vi "STAGE+mono+counter_edit18.vi"() -> ()   [LabVIEW 2017]
panel:
  out "Array 3":dbl[][](array[numeric])
  out "Array 2":dbl[](array[numeric])
  out "XY Graph 2":cluster{dbl[], dbl[]}[](graph)
  out "Waveform Graph":waveform(dbl)[](graph)
  out "XY Graph":cluster{dbl[], dbl[]}(graph)
  out "PROGRESS":u8(slide) max=10 step=10 scale=0.0..5.0
  in  "?":enum32{"DELAY", "COUNTER", "MONO", "PLOT"}(tab)
  out "Final time [ps]":dbl
  out "Current time [ps]":dbl
  out "Initial time [ps]":dbl
  in  "Set this as t0":bool
  in  "Axis":i32=1
  in  "Motor ON":bool
  in  "Motor OFF":bool
  out "Current Position [mm]":dbl
  out "Final Position [mm]":dbl
  in  "Data Points":i32=100
  out "Current Point":i32
  in  "Step Size [um]":i32=10
  in  "Target [mm]":dbl format="%.3f"
  in  "Move":bool
  out "Initial position [mm]":dbl
  in  "GPIB address":string="23"
  in  "Count Mode":u16(ring) items=["A,B for Preset T", "A-B for Preset T", "A+B for Preset T", "A for Preset B"]
  in  "Trigger mode":u16(ring) items=["10 MHz"=0, "Input 2"=2, "Input T"=3]
  in  "Channel A Input":u16(ring)=1 items=["10 MHz", "Input 1"]
  in  "Channel B Input":u16(ring)=2 items=["Input 1"=1, "Input 2"=2]
  in  "Number of Measurements\n to take at one point/ Number of Periods":u16=1 min=1 max=2000 step=1
  in  "Time between measurements\n at one point (s)/Dwell Time":dbl=0.002 min=0.002 max=60.0 step=0.001
  in  "gate mode (CW:0)":i16(slide) scale=0.0..2.0 scale format="%.2f"
  out "Counts":i32
  in  "Integrating time \nin 10^-7 sec":dbl=10000000.0
  in  "Discriminator Level (mV)":dbl min=-300.0 max=300.0 step=0.2
  in  "Discriminator Slope":bool
  in  "Channel":i16 min=0 max=2 step=1
  out "Grating #":dbl
  out "Blaze angle":dbl
  out "Grooves/mm":dbl
  out "Mono port":T1(ring)
  out "Time delay":u32=450000 min=1
  in  "Step size":dbl=10.0 min=0.0
  in  "Scan to":i32=4000
  in  "Scan from":i32=2600
  out "Current wavelength":dbl
  in  "?":bool
  in  "Array":dbl[](array[numeric])
  out "Numeric":i32
  out "Numeric 2":i32
  out "Timeout 2":bool
  in  "?":bool
  out "Timeout":bool
  in  "Collect Data!":bool
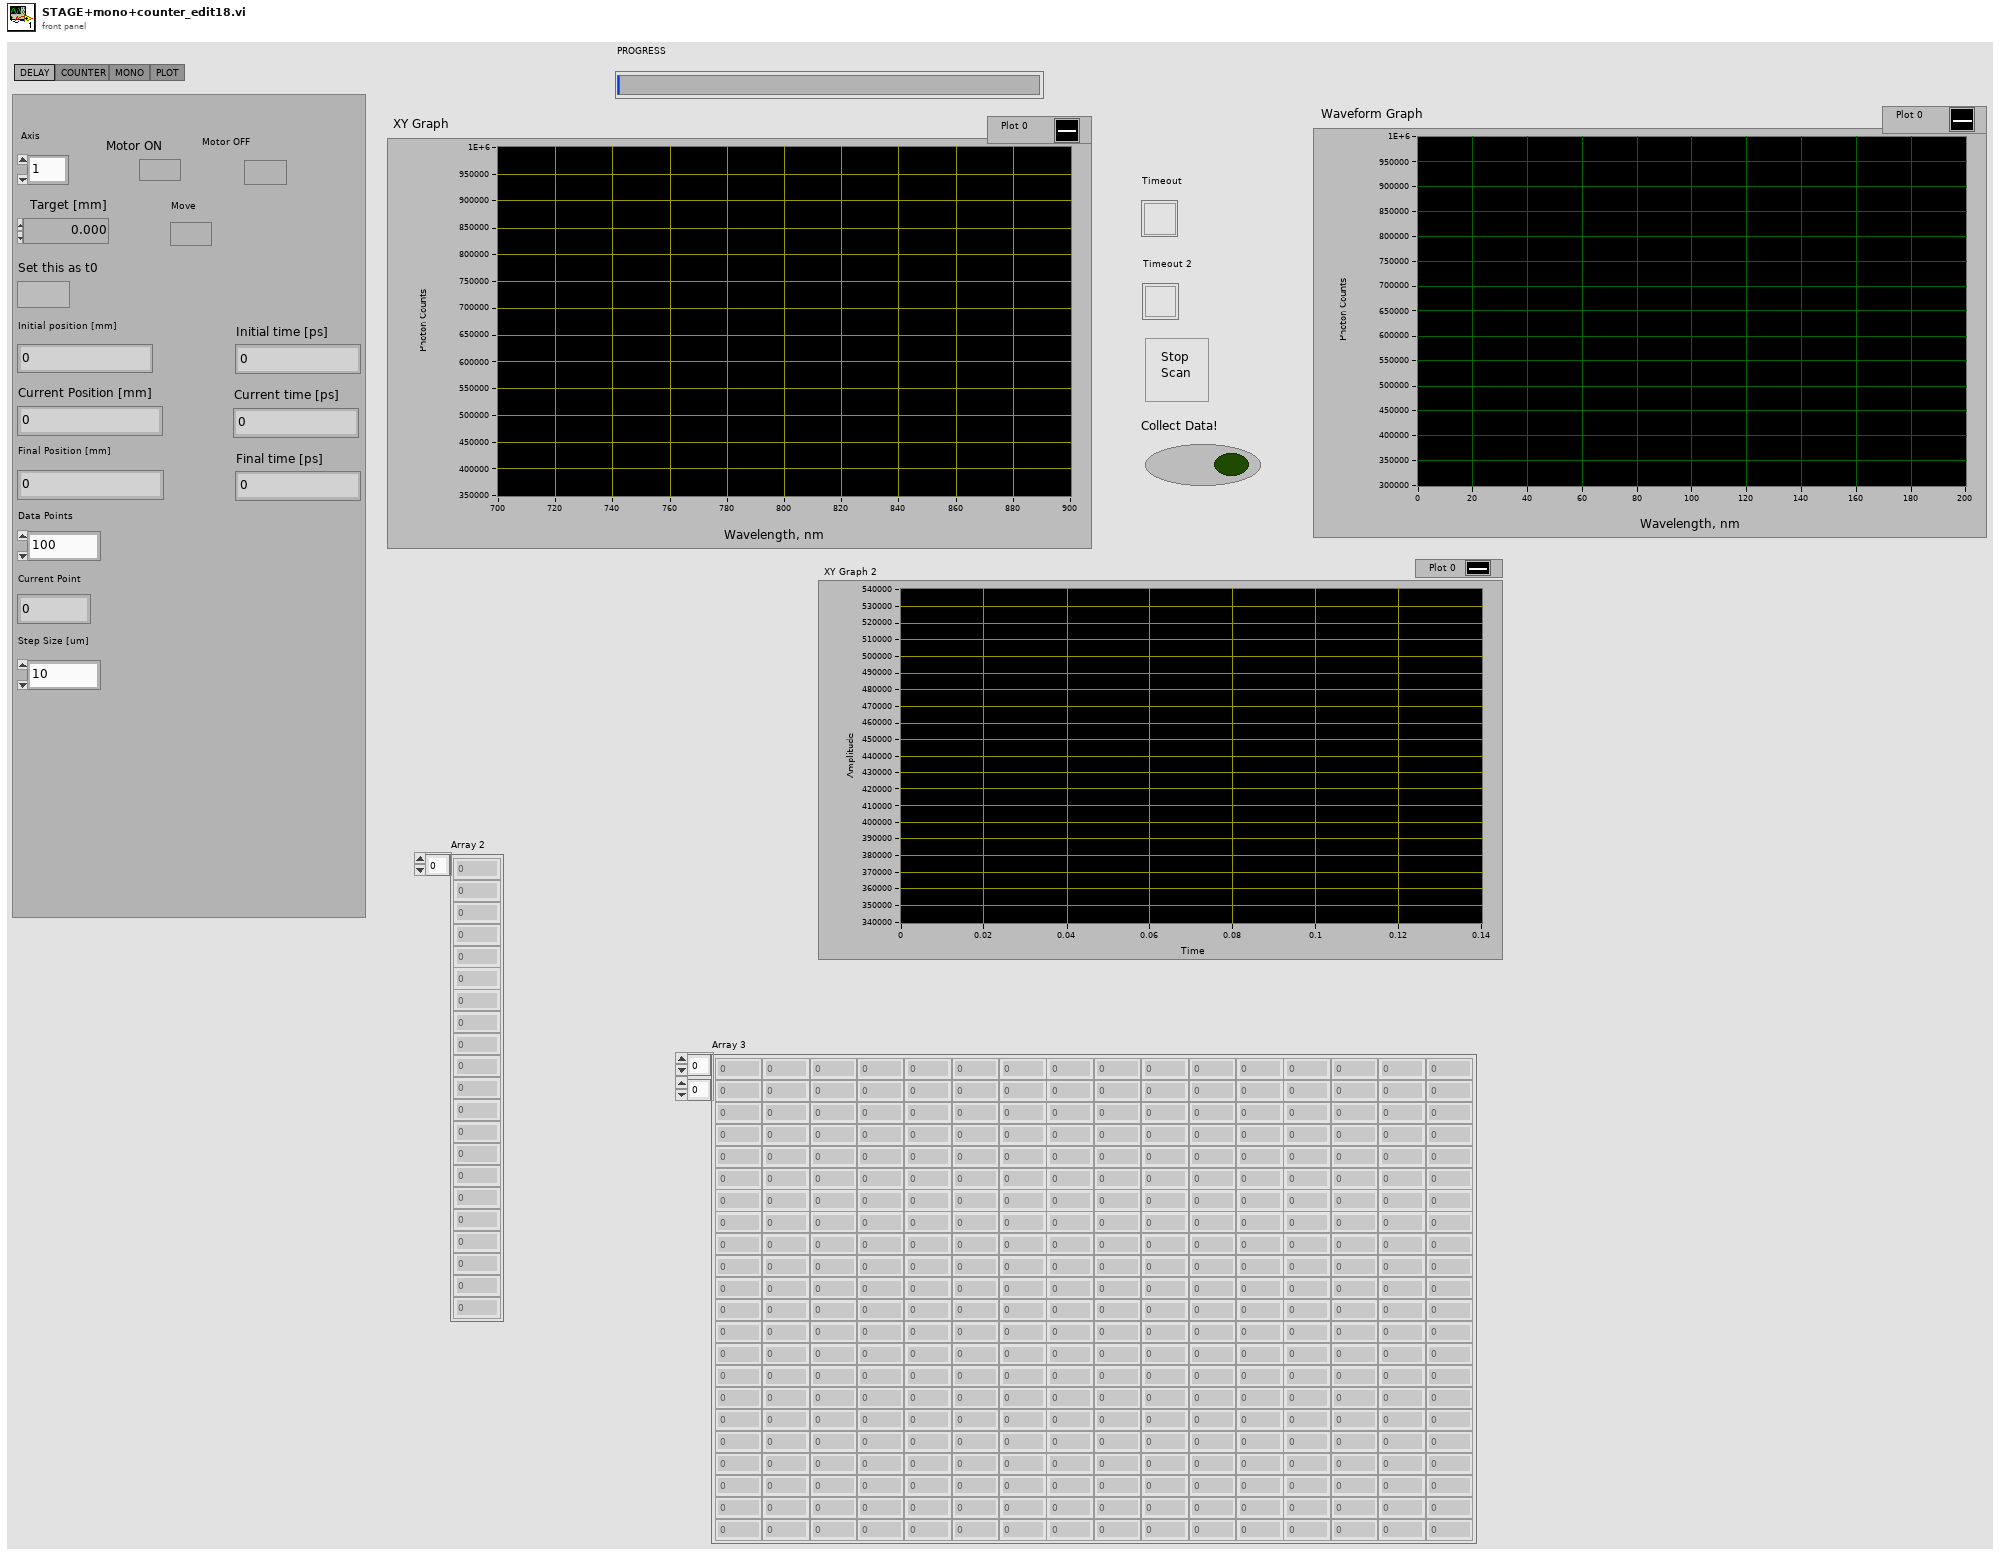
[diagram p1: front panel]
types:
  T1 = enum8{"COM 1", "COM 2", "COM 3", "COM 4", "COM 5", "COM 6", "COM 7", "COM 8", "COM 9"}
  T2 = cluster{"input XON/XOFF":bool, "input HW Handshake":bool, "input alt HW HShk":bool, "output XON/XOFF":bool, "output HW Handshake":bool, "output alt HW HShk":bool, "XOFF byte":u8, "XON byte":u8, "parity error byte":u16}
  T3 = enum16{"no parity", "odd parity", "even parity", "mark parity", "space parity"}
  T4 = typedef "NI_Matrix.lvlib/RealMatrix.ctl" = dbl[][]
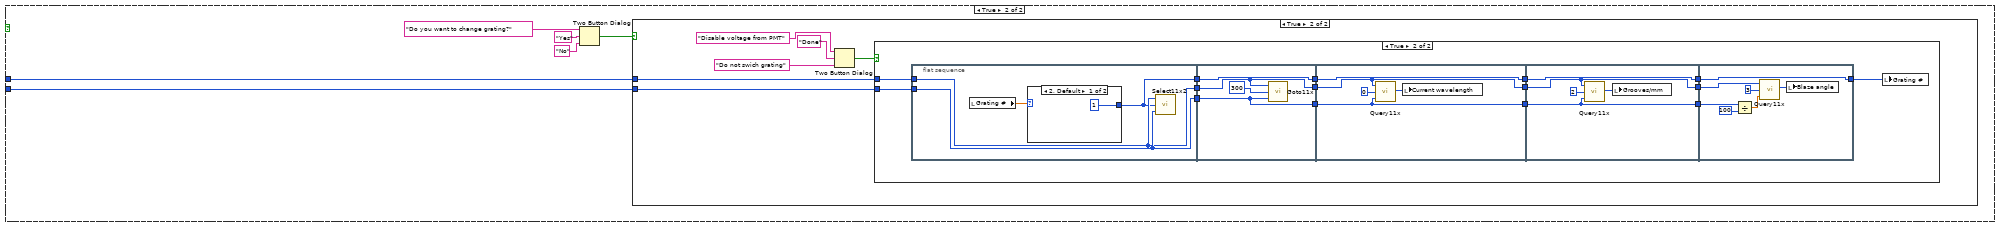
[diagram p2: hidden frame]
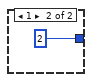
[diagram p5: hidden frame]
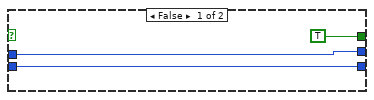
[diagram p6: hidden frame]
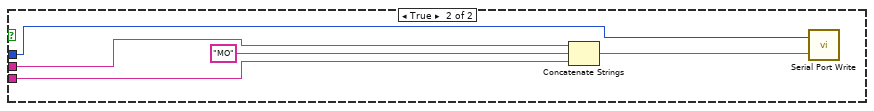
[diagram p7: hidden frame]
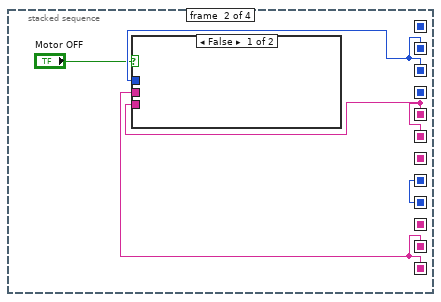
[diagram p8: hidden frame]
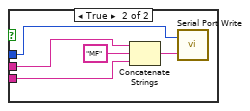
[diagram p9: hidden frame]
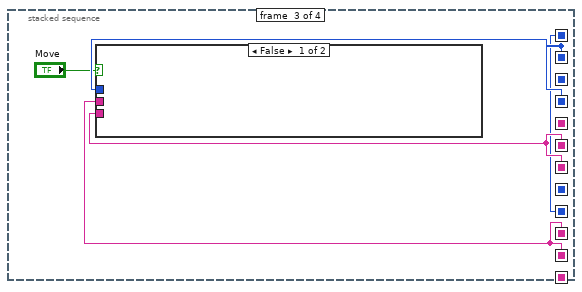
[diagram p10: hidden frame]
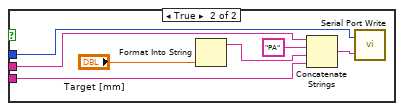
[diagram p11: hidden frame]
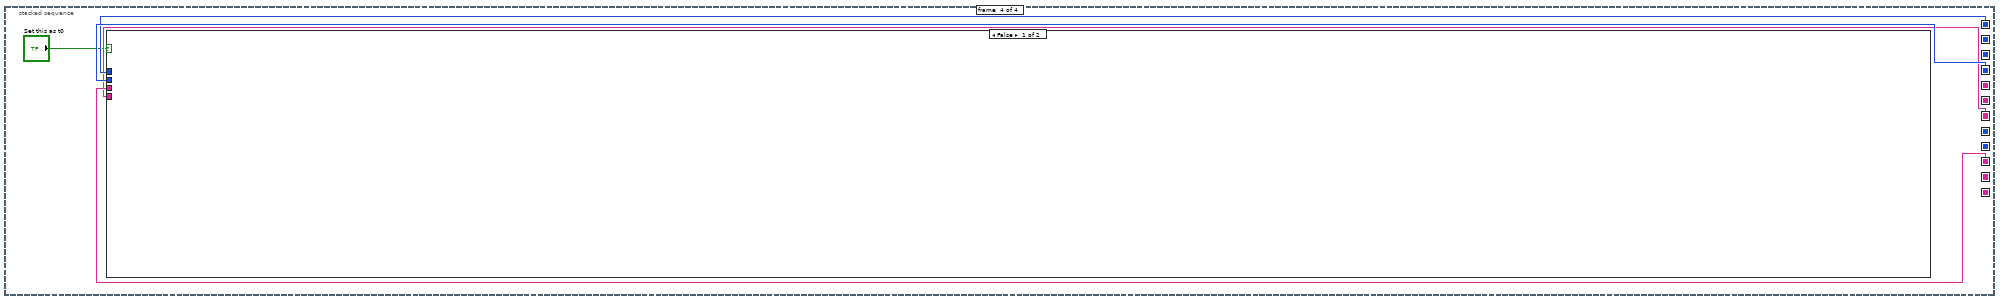
[diagram p12: hidden frame]
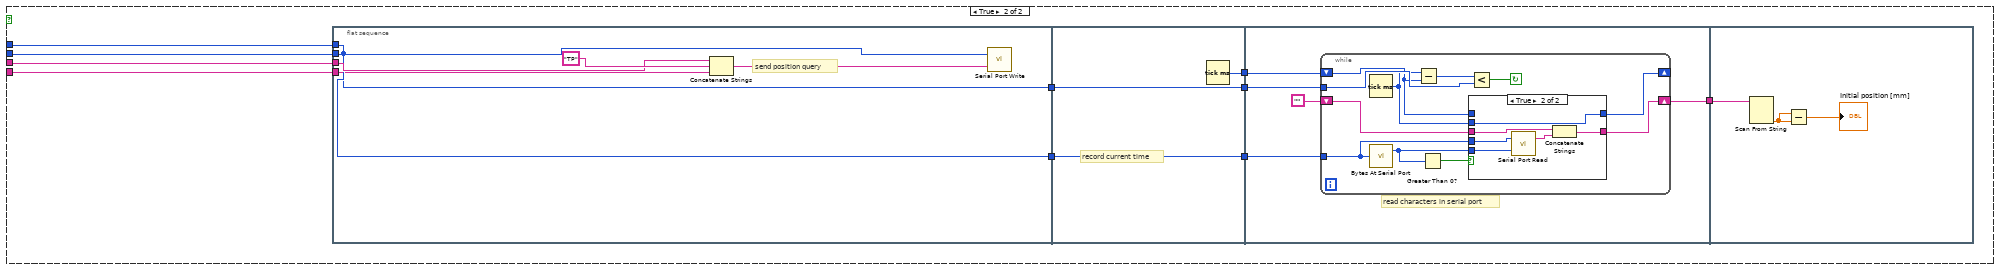
[diagram p13: hidden frame]
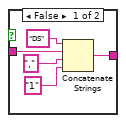
[diagram p15: hidden frame]
diagram:
  (unwired) FALSE
  w41 = u32 19200  # baud rate
  w40 = u16 8  # data bits
  w39 = enum16{"1 bit", "1.5 bits", "2 bits"}."1 bit"  # stop bits
  w43 = T3."no parity"  # parity
  w38 = 4  # 0=COM1 so n=COM(n+1)
  w42 = u16 1024  # buffer size
  n1 = flat-sequence {
    tunnel: ["Data Points"] -> w47
    tunnel: "Axis" -> [w69]
    tunnel: [w61] -> w46
    tunnel: [w69] -> w45
    tunnel: ["Step Size [um]"] -> w19
    tunnel: [w61] -> w18
    tunnel: ["Step Size [um]"] -> w17
    tunnel: ["Data Points"] -> w16
    tunnel: [w61] -> w15
    tunnel: [w60] -> w14
    tunnel: [w61] -> w12
    tunnel: [w60] -> w11
    tunnel: [w63] -> w10
    tunnel: [w52] -> w9
    tunnel: [w53] -> w2
    tunnel: [w52] -> w1
    tunnel: w47 -> [w158]
    tunnel: w46 -> [w157]
    tunnel: w45 -> [w156]
    tunnel: w38 -> [w152]
    tunnel: "GPIB address" -> [w151]
    tunnel: "GPIB address" -> [w150]
    tunnel: w19 -> [w139]
    tunnel: w18 -> [w137]
    tunnel: w17 -> [w136]
    tunnel: w16 -> [w134]
    tunnel: w15 -> [w129]
    tunnel: w14 -> [w128]
    tunnel: "Integrating time \nin 10^-7 sec" -> [w127]
    tunnel: w12 -> [w125]
    tunnel: w11 -> [w124]
    tunnel: w10 -> [w123]
    tunnel: w9 -> [w121]
    tunnel: w5 -> [w111]
    tunnel: w4 -> [w110]
    tunnel: w3 -> [w109]
    tunnel: w2 -> [w77]
    tunnel: w1 -> [w76]
    frame #0 {
      n2 = while {
        stop <- "Collect Data!" stop-if-true
        n3 = Multiply(x=1, y=1000) -> (x*y=w51:i32)
        n4 = Wait (ms)(milliseconds to wait=w51) -> ()  [unwired: 1 out]
      }
    }
    frame #1 {
      w54 = 1000000000000.0
      w59 = 1000
      w62 = 300000000
      w64 = 1000
      n5 = local read "Initial position [mm]"() -> (w61:dbl)
      n6 = Multiply(x="Step Size [um]", y="Data Points") -> (x*y=w68:i32)
      n7 = Divide(x="Step Size [um]", y=w64) -> (x/y=w63:dbl)
      n8 = Divide(x=w68, y=w64) -> (x/y=w67:dbl)
      n9 = Add(x=w61, y=w67) -> (x+y=w60:dbl)
      "Final Position [mm]" <- w60
      n10 = Divide(x=w60, y=w59) -> (x/y=w58:dbl)
      n11 = Divide(x=w61, y=w59) -> (x/y=w57:dbl)
      n12 = Divide(x=w58, y=w62) -> (x/y=w55:dbl)
      n13 = Divide(x=w57, y=w62) -> (x/y=w56:dbl)
      n14 = Multiply(x=w55, y=w54) -> (x*y=w53:dbl)
      "Final time [ps]" <- w53
      n15 = Multiply(x=w56, y=w54) -> (x*y=w52:dbl)
      "Initial time [ps]" <- w52
    }
    frame #2 {
      w91 = "\r\n"
      n16 = Increment(x=w134) -> (x+1=w135:i32)
      n17 = Divide(x=w139, y=1000.0) -> (x/y=w115:dbl)
      n18 = for {
        N: w135 -> [_]
        tunnel: w115 -> [w169]
        tunnel: w137 -> [w167]
        tunnel: [w160] -> w133 mode=indexing
        i -> [w168]
        # "distances"
        n19 = Multiply(x=w169, y=w168) -> (x*y=w166:dbl)
        n20 = Add(x=w167, y=w166) -> (x+y=w165:dbl)
        n21 = Divide(x=w165, y=1000) -> (x/y=w159:dbl)
        n22 = Divide(x=w159, y=300000000) -> (x/y=w162:dbl)
        n23 = Multiply(x=w162, y=1000000000000.0) -> (x*y=w160:dbl)
      }
      n24 = To Time Stamp(1:"Scan from") -> (0:w82:timestamp)
      n25 = Multiply(x="Scan to", y=1) -> (x*y=w122:i32)
      n26 = Multiply(x=1, y="Scan from") -> (x*y=w114:i32)
      n27 = Divide(x=w115, y=1000.0) -> (x/y=w116:dbl)
      n28 = Subtract(x=w122, y=w114) -> (x-y=w145:i32)
      n29 = Divide(x=w145, y="Step size") -> (x/y=w144:dbl)
      n30 = Divide(x=w116, y=300000000) -> (x/y=w118:dbl)
      n31 = Bundle By Name("Y"=dbl[] [], "t0"=w82, "dt"="Step size") -> (w79:waveform(dbl))  [unwired: 1 in]
      n32 = local read "Numeric"() -> (w71:i32)
      n33 = Multiply(x=w118, y=1000000000000.0) -> (x*y=w75:dbl)
      n34 = local read "Numeric 2"() -> (w72:i32)
      n35 = Build Array(w79) -> (w78:waveform(dbl)[])
      n36 = Round Toward -Infinity(1:w144) -> (0:w143:dbl)
      n37 = Concatenate Strings("\r", "\n") -> (w153:string)
      n38 = property on="XY Graph 2" class="XYGraph (strict)"("XScale.Increment"=w75, "XScale.Maximum"=w77, "XScale.Minimum"=w76) -> ()  [unwired: 2 in, 2 out]
      n39 = Initialize Array(0.0, w71, w72) -> ()  [unwired: 1 out]
      n40 = Increment(x=w143) -> (x+1=w113:dbl)
      n41 = for {
        N: w158 -> [w184]
        tunnel: w157 -> [w247]
        tunnel: w136 -> [w243]
        tunnel: w156 -> [w240]
        tunnel: w153 -> [w237]
        tunnel: w152 -> [w238]
        tunnel: w151 -> [w236]
        tunnel: w110 -> [w233]
        tunnel: w111 -> [w235]
        tunnel: w150 -> [w234]
        tunnel: [w194] -> w84 mode=indexing
        tunnel: w114 -> [w228]
        tunnel: "Step size" -> [w227]
        tunnel: w143 -> [w226]
        tunnel: w129 -> [_]
        tunnel: w128 -> [_]
        tunnel: w127 -> [w225]
        tunnel: "Scan to" -> [w224]
        tunnel: "Scan from" -> [w223]
        tunnel: "Step size" -> [w200]
        tunnel: w125 -> [w216]
        tunnel: w124 -> [w214]
        tunnel: w123 -> [w217]
        tunnel: w75 -> [w186]
        tunnel: w121 -> [w221]
        tunnel: "Scan from" -> [w201]
        tunnel: "Step size" -> [w202]
        shift-right: [w185] -> _
        shift-left: dbl[] [] -> [w180]
        tunnel: w111 -> [w199]
        tunnel: w110 -> [w198]
        tunnel: w109 -> [w197]
        shift-right: [w191] -> _
        shift-left: w78 -> [w192]
        shift-right: [w178] -> _
        shift-left: dbl[][] [] -> [w177]
        i -> [w183]
        w196 = dbl[] []
        w215 = 1000
        w218 = 300000000
        n42 = To Time Stamp(1:w228) -> ()  [unwired: 1 out]
        n43 = property on="PROGRESS" class="Slide (strict)"("Scale.Increment"=1, "Scale.Maximum"=w184, "Scale.Minimum"=0) -> ()  [unwired: 2 in, 2 out]
        n44 = flat-sequence {
          tunnel: w236 -> [w273]
          tunnel: w235 -> [w272]
          tunnel: w233 -> [w271]
          tunnel: w228 -> [w270]
          tunnel: w227 -> [w269]
          tunnel: w226 -> [w268]
          tunnel: w224 -> [w267]
          tunnel: w223 -> [w266]
          tunnel: w196 -> [w265]
          tunnel: w196 -> [w264]
          tunnel: w202 -> [w263]
          tunnel: w201 -> [w262]
          tunnel: w200 -> [w261]
          tunnel: w199 -> [w260]
          tunnel: w198 -> [w259]
          tunnel: w197 -> [w258]
          tunnel: [w256] -> w195
          tunnel: [w257] -> _
          tunnel: [w256] -> w193
          tunnel: [w438] -> w194
          tunnel: w195 -> [w438]
          tunnel: [w437] -> w179
          tunnel: [w436] -> w176
          frame #0 {
            # "step size"
            n45 = while {
              tunnel: w271 -> [_]
              tunnel: w272 -> [_]
              tunnel: w273 -> [w279]
              tunnel: w270 -> [w307]
              tunnel: w269 -> [w306]
              tunnel: w268 -> [w305]
              tunnel: w267 -> [w275]
              tunnel: w266 -> [w274]
              tunnel: w261 -> [w276]
              tunnel: w263 -> [w303]
              shift-right: [w299] -> w256
              shift-left: w264 -> [w298]
              shift-right: [w293] -> w257
              shift-left: w265 -> [w301]
              tunnel: w262 -> [w296]
              tunnel: w260 -> [w283]
              tunnel: w259 -> [w282]
              tunnel: w258 -> [w281]
              i -> [w304]
              stop <- w310 stop-if-true
              n46 = property on="XY Graph" class="XYGraph (strict)"("XScale.Increment"=w276, "XScale.Maximum"=w275, "XScale.Minimum"=w274) -> ()  [unwired: 2 in, 2 out]
              n47 = Multiply(x=w304, y=w306) -> (x*y=w311:dbl)
              n48 = Multiply(x=w304, y=w303) -> (x*y=w302:dbl)
              n49 = Greater Or Equal?(x=w304, y=w305) -> (x >= y?=w308:bool)
              n50 = Add(x=w302, y=w296) -> ()  [unwired: 1 out]
              n51 = Add(x=w311, y=w307) -> (x+y=w280:dbl)
              n52 = Or(x="?", y=w308) -> (x .or. y?=w310:bool)
              n53 = Build Array (concatenate)(w301, w280) -> (w300:dbl[])
              n54 = flat-sequence {
                tunnel: w279 -> [w326]
                tunnel: w280 -> [w327]
                tunnel: [w327] -> w287
                tunnel: [w313] -> w286
                tunnel: [w312] -> w285
                tunnel: [w326] -> w284
                tunnel: w283 -> [w316]
                tunnel: w282 -> [w315]
                tunnel: w281 -> [w314]
                tunnel: [w360] -> w292
                tunnel: [w359] -> w291
                tunnel: [w357] -> w290
                tunnel: w287 -> [w361]
                tunnel: w286 -> [w360]
                tunnel: w285 -> [w359]
                tunnel: w284 -> [w357]
                tunnel: w292 -> [w368]
                tunnel: w291 -> [w367]
                tunnel: w290 -> [w362]
                tunnel: [w362] -> w278
                tunnel: w278 -> [w370]
                tunnel: [w370] -> w277
                tunnel: w277 -> [w423]
                tunnel: [w423] -> w289
                tunnel: w289 -> [w424]
                tunnel: [w424] -> w288
                tunnel: [w430] -> w295
                tunnel: w288 -> [w431]
                frame #0 {
                  n55 = flat-sequence {
                    tunnel: w316 -> [w333]
                    tunnel: [w333] -> w325
                    tunnel: w315 -> [w335]
                    tunnel: [w335] -> w324
                    tunnel: w314 -> [w331]
                    tunnel: [w331] -> w323
                    tunnel: w325 -> [w339]
                    tunnel: [w339] -> w322
                    tunnel: w324 -> [w340]
                    tunnel: [w340] -> w321
                    tunnel: w323 -> [w337]
                    tunnel: [w337] -> w320
                    tunnel: w322 -> [w348]
                    tunnel: [w348] -> w319
                    tunnel: w321 -> [w345]
                    tunnel: [w345] -> w318
                    tunnel: w320 -> [w343]
                    tunnel: [w343] -> w317
                    tunnel: w319 -> [w350]
                    tunnel: w318 -> [w351]
                    tunnel: w317 -> [_]
                    tunnel: [w351] -> w313
                    tunnel: [w350] -> w312
                    frame #0 {
                      n56 = call "Query11x.vi"("port number"=w335, "QUERY"=u16 0, "time delay"=w333) -> ("timeout"=w332:bool, "STATUS MESSAGE"=w330:u16)  [unwired: 2 out]
                      n57 = local write "Timeout"(w332) -> ()
                      n58 = Divide(x=w330, y=1 ("Numeric")) -> (x/y=→"Current wavelength":dbl)
                    }
                    frame #1 {
                      n59 = call "Query11x.vi"("port number"=w340, "QUERY"=u16 2, "time delay"=w339) -> ("timeout"=w338:bool, "STATUS MESSAGE"=→"Grooves/mm":u16)  [unwired: 2 out]
                      n60 = local write "Timeout"(w338) -> ()
                    }
                    frame #2 {
                      n61 = Divide(x=w348, y=i16 100 ("device (1)")) -> (x/y=w346:dbl)
                      n62 = call "Query11x.vi"("port number"=w345, "QUERY"=u16 3, "time delay"=w346) -> ("timeout"=w344:bool, "STATUS MESSAGE"=→"Blaze angle":u16)  [unwired: 2 out]
                      n63 = local write "Timeout"(w344) -> ()
                    }
                    frame #3 {
                      n64 = Divide(x=w350, y=i16 100 ("device (1)")) -> (x/y=w354:dbl)
                      n65 = call "Query11x.vi"("port number"=w351, "QUERY"=u16 4, "time delay"=w354) -> ("timeout"=w353:bool, "STATUS MESSAGE"=→"Grating #":u16)  [unwired: 2 out]
                      n66 = local write "Timeout"(w353) -> ()
                    }
                  }
                }
                frame #1 {
                  n67 = call "Goto11x.vi"("time delay"=w359, "WAVELENGTH"=w361, "port number"=w360) -> ("timeout"=w358:bool)  [unwired: 2 out]
                  n68 = local write "Timeout 2"(w358) -> ()
                }
                frame #2 {
                  # "set counter time in 10^-7 seconds in CW"
                  n69 = call "Query11x.vi"("port number"=w368, "QUERY"=0, "time delay"=w367) -> ("timeout"=w366:bool, "STATUS MESSAGE"=w365:u16)  [unwired: 2 out]
                  n70 = local write "Timeout 2"(w366) -> ()
                  n71 = Divide(x=w365, y=1) -> (x/y=w364:dbl)
                  n72 = local write "Current wavelength"(w364) -> ()
                }
                frame #3 {
                  # "Configures discriminator."
                  n73 = flat-sequence {
                    tunnel: w370 -> [w380]
                    tunnel: [w380] -> w379
                    tunnel: [w387] -> w378
                    tunnel: [w385] -> w377
                    tunnel: "Discriminator Slope" -> [w386]
                    tunnel: w379 -> [w385]
                    tunnel: w371 -> [w384]
                    tunnel: w378 -> [w406]
                    tunnel: [w407] -> w376
                    tunnel: w377 -> [w405]
                    tunnel: [w405] -> w375
                    tunnel: w371 -> [w403]
                    tunnel: w376 -> [w419]
                    tunnel: w375 -> [w418]
                    tunnel: "Discriminator Level (mV)" -> [w413]
                    tunnel: w371 -> [w412]
                    frame #0 {
                      # "Flush I/O buffers."
                      n74 = for {
                        N: 5 -> [_]
                        tunnel: w380 -> [w382]
                        n75 = GPIB Write(0:w382, 1:"\r") -> ()  [unwired: 3 in, 2 out]
                      }
                    }
                    frame #1 {
                      # "Set discriminator slope."
                      n76 = case shown="True" w386 {
                        tunnel: [w393 w398] -> w388
                        tunnel: w384 -> [w392 w397]
                        frame False {
                          n77 = Concatenate Strings("DS", w392, ",", "1") -> (w393:string)
                        }
                        frame True {
                          n78 = Concatenate Strings("DS", w397, ",", "0") -> (w398:string)
                        }
                      }
                      n79 = GPIB Write(0:w385, 1:w388, 2:5) -> (6:w387:errorcluster)  [unwired: 2 in, 1 out]
                    }
                    frame #2 {
                      # "Set discriminator mode to fixed."
                      n80 = Concatenate Strings("DM", w403, ",", "0") -> (w402:string)
                      n81 = GPIB Write(0:w405, 1:w402, 2:5, 3:w406) -> (6:w407:errorcluster)  [unwired: 1 in, 1 out]
                    }
                    frame #3 {
                      # "Set discriminator level.\nMust be between +300 and -300 mV."
                      n82 = Divide(x=w413, y=1000.0) -> (x/y=w421:dbl)
                      n83 = Number To Fractional String(number=w421, precision (6)=i16 4) -> (F-format string=w410:string)  [unwired: 2 in]
                      n84 = Concatenate Strings("DL", w412, ",", w410) -> (w417:string)
                      n85 = GPIB Write(0:w418, 1:w417, 2:5, 3:w419) -> (6:w414:errorcluster)  [unwired: 1 in, 1 out]
                      n86 = call <vilib>:"General Error Handler.vi"("type of dialog (OK msg:1)"=1, "error in (no error)"=w414) -> ()  [unwired: 9 in, 5 out]
                    }
                  }
                  n87 = Number To Decimal String(number="Channel") -> (decimal integer string=w371:string)  [unwired: 1 in]
                }
                frame #4 {
                  n88 = call "Start.vi"("GPIB Address"=w423) -> ()  [unwired: 9 in]
                }
                frame #5 {
                  # "Wait for Scan to Finish"
                  n89 = for {
                    N: 1 -> [_]
                    tunnel: w424 -> [w426]
                    n90 = while {
                      tunnel: w426 -> [w427]
                      stop <- w429 stop-if-true
                      n91 = call "ScanDone.vi"("Wait (ms)"=1000, "GPIB Address"=w427) -> ("Scan Finished?"=w429:bool)
                    }
                  }
                }
                frame #6 {
                  n92 = call "Read Data.vi"("Channel Number"=0, "GPIB Address"=w431, "Number of Datapoints"=1) -> ("Data"=w432:i32[])
                  n93 = Index Array(array=w432, index=0) -> (element=w430:i32)
                  "Counts" <- w430
                }
              }
              n94 = Build Array (concatenate)(w298, w295) -> (w297:dbl[])
              n95 = Bundle(w300, w297) -> (w294:cluster{dbl[], dbl[]})  [unwired: 1 in]
              "XY Graph" <- w294
              n96 = Unbundle(w294) -> (w293:dbl[], w299:dbl[])
            }
          }
          frame #1 {
            n97 = Array Size(array="Array") -> (size(s)=w436:i32)
            n98 = flat-sequence {
              tunnel: w438 -> [w444]
              tunnel: "Array" -> [w443]
              tunnel: w436 -> [w442]
              tunnel: [w440] -> w437
              frame #0 {
                n99 = for {
                  N: w442 -> [w449]
                  tunnel: w443 -> [w456]
                  tunnel: w444 -> [w451]
                  shift-right: [w445] -> w440
                  shift-left: dbl[] [] -> [w446]
                  i -> [w448]
                  n100 = local read "Scan from"() -> (w454:i32)
                  n101 = Index Array(array=w456, index=w448) -> (element=w455:dbl)
                  n102 = local read "Step size"() -> (w452:dbl)
                  n103 = Subtract(x=w455, y=w454) -> (x-y=w453:dbl)
                  n104 = Divide(x=w453, y=w452) -> (x/y=w450:dbl)
                  n105 = Index Array(array=w451, index=w450) -> (element=w447:dbl)
                  n106 = Insert Into Array(array=w446, index=w448, new element=w447) -> (w445:dbl[])
                  "Numeric" <- w449
                }
              }
            }
          }
        }
        n107 = stacked-sequence {
          tunnel: w233 -> [w458]
          tunnel: w234 -> [_]
          frame #0 {
            n108 = call <vilib>:"Close Serial Driver.vi"("port number"=w458) -> ()  [unwired: 1 out]
            n109 = GPIB Misc(0:"loc 23" ("command string")) -> ()  [unwired: 1 in, 3 out]
          }
        }
        n110 = Divide(x=w217, y=w215) -> (x/y=w213:dbl)
        n111 = Divide(x=w214, y=w215) -> (x/y=w211:dbl)
        n112 = Divide(x=w216, y=w215) -> (x/y=w212:dbl)
        n113 = Multiply(x=w186, y=w183) -> (x*y=w222:dbl)
        n114 = Number To Decimal String(number=w225) -> (decimal integer string=w231:string)  [unwired: 1 in]
        n115 = Add(x=1, y=w183) -> (x+y=→"PROGRESS":i32)
        n116 = Divide(x=w243, y=1000) -> (x/y=w242:dbl)
        n117 = Divide(x=w213, y=w218) -> (x/y=w207:dbl)
        n118 = Divide(x=w211, y=w218) -> (x/y=w205:dbl)
        n119 = Divide(x=w212, y=w218) -> (x/y=w206:dbl)
        n120 = Add(x=w221, y=w222) -> (x+y=w181:dbl)
        n121 = Concatenate Strings("CP 2,", w231) -> (w229:string)
        n122 = Multiply(x=w207, y=1000000000000.0) -> ()  [unwired: 1 out]
        n123 = Multiply(x=w205, y=1000000000000.0) -> ()  [unwired: 1 out]
        n124 = Multiply(x=w206, y=1000000000000.0) -> ()  [unwired: 1 out]
        n125 = Multiply(x=w242, y=w183) -> (x*y=w246:dbl)
        n126 = Add(x=w247, y=w246) -> (x+y=w245:dbl)
        n127 = Format Into String(w240) -> (resulting string=w239:string)  [unwired: 3 in, 1 out]
        n128 = GPIB Write(0:w236, 1:w229, 2:i16 5 ("mode (0)")) -> ()  [unwired: 2 in, 2 out]
        n129 = Build Array (concatenate)(w180, w181) -> (w182:dbl[])
        n130 = flat-sequence {
          tunnel: w245 -> [w461]
          tunnel: [w461] -> w241
          tunnel: w237 -> [w463]
          tunnel: w239 -> [w462]
          tunnel: w238 -> [w459]
          tunnel: w241 -> [w472]
          frame #0 {
            n131 = Format Into String(w461) -> (resulting string=w460:string)  [unwired: 3 in, 1 out]
            n132 = Wait (ms)(milliseconds to wait=u32 100) -> ()  [unwired: 1 out]
            n133 = Concatenate Strings(w462, "PA" ("Substring"), w460, w463) -> (w465:string)
            n134 = call <vilib>:"Serial Port Write.vi"("string to write"=w465, "port number"=w459) -> ()  [unwired: 1 out]
          }
          frame #1 {
            n135 = Divide(x=w472, y=1000) -> (x/y=w470:dbl)
            n136 = Wait (ms)(milliseconds to wait=u32 1000) -> ()  [unwired: 1 out]
            n137 = Divide(x=w470, y=300000000) -> (x/y=w469:dbl)
            n138 = Multiply(x=w469, y=1000000000000.0) -> (x*y=→"Current time [ps]":dbl)
            "Current Position [mm]" <- w472
          }
        }
        n139 = local read "Scan from"() -> (w189:i32)
        n140 = local read "Step size"() -> (w187:dbl)
        n141 = To Time Stamp(1:w189) -> (0:w188:timestamp)
        n142 = Bundle By Name("Y"=w193, "t0"=w188, "dt"=w187) -> (w190:waveform(dbl))  [unwired: 1 in]
        n143 = Build Array (concatenate)(w192, w190) -> (w191:waveform(dbl)[])
        "Waveform Graph" <- w191
        n144 = for {
          N: w176 -> [_]
          tunnel: [w255] -> w185
          tunnel: w182 -> [w254]
          tunnel: w179 -> [w252]
          tunnel: [w251] -> w178
          tunnel: w177 -> [w253]
          tunnel: [w248] -> w175 mode=indexing
          i -> [w250]
          n145 = Build Array (concatenate)(w253, w252) -> (w251:dbl[][])
          "Array 3" <- w251
          n146 = Index Array(array=w251, index (col)=w250) -> (element=w249:dbl[])  [unwired: 1 in]
          n147 = Bundle(w254, w249) -> (w248:cluster{dbl[], dbl[]})  [unwired: 1 in]
          n148 = Unbundle(w248) -> (w255:dbl[])  [unwired: 1 out]
          n149 = Index Array(array=w252, index=w250) -> ()  [unwired: 1 out]
          "Array 2" <- w254
        }
        "XY Graph 2" <- w175
        "Current Point" <- w183
        "Numeric 2" <- w184
      }
      n150 = for {
        N: w113 -> [_]
        tunnel: "Step size" -> [w174]
        tunnel: w114 -> [w172]
        tunnel: [w170] -> w112 mode=indexing
        i -> [w173]
        # "wavelengths"
        n151 = Multiply(x=w174, y=w173) -> (x*y=w171:dbl)
        n152 = Add(x=w172, y=w171) -> (x+y=w170:dbl)
      }
      n153 = Build Array (concatenate)(0, w133) -> (w85:dbl[])
      n154 = Build Array(w112) -> (w142:dbl[][])
      n155 = local read "Integrating time \nin 10^-7 sec"() -> (w89:dbl)
      n156 = Transpose Matrix(1:w142) -> (0:w141:dbl[][])
      n157 = Transpose Matrix(1:w84) -> (0:w140:dbl[][])
      n158 = Build Array (concatenate)(w141, w140) -> (w86:T4)
      n159 = Insert Into Array(array=w86, index (row)=0, new element=w85) -> (w130:T4)  [unwired: 1 in]
      n160 = local read "Blaze angle"() -> (w108:dbl)
      n161 = local read "Grating #"() -> (w107:dbl)
      n162 = Multiply(x=w89, y=1e-07) -> (x*y=w88:dbl)
      n163 = Get Date/Time In Seconds() -> (seconds since 1Jan1904=w101:timestamp)
      n164 = Array To Spreadsheet String(delimiter (Tab)=",", array=w130, 3:"%f" ("format string")) -> (spreadsheet string=w90:string)
      n165 = Format Date/Time String(time format string (%c)="%Y-%b-%d %H:%M:%S", seconds (now)=w101) -> (date/time string=w102:string)  [unwired: 1 in]
      n166 = Number To Decimal String(number=w88) -> (decimal integer string=w103:string)  [unwired: 1 in]
      n167 = Number To Decimal String(number=w107) -> (decimal integer string=w104:string)  [unwired: 1 in]
      n168 = Number To Decimal String(number=w108) -> (decimal integer string=w92:string)  [unwired: 1 in]
      n169 = call <vilib>:"Space Constant.vi"() -> ("String"=w105:string)
      n170 = Concatenate Strings(w91, "Data was taken on ", w102, w91, "Integration Time is ", w103, w105, "s", w91, "Monochromator gratng # ", w104, "; ", "blazed for ", w92, w105, "nm", w91, w91, w91, w90) -> (w106:string)
      n171 = Write to Text File(text=w106) -> ()  [unwired: 3 in, 3 out]
    }
  }
  n172 = flat-sequence {
    tunnel: [w476] -> w32
    tunnel: [w475] -> w31
    frame #0 {
      n173 = call "CM Com Read ini.vi"() -> ("Mono port"=w475:T1, "time delay1"=w476:u32)  [unwired: 7 in]
    }
  }
  n174 = call <vilib>:"Serial Port Init.vi"("flow control etc."=T2 {"input XON/XOFF"=FALSE, "input HW Handshake"=FALSE, "input alt HW HShk"=FALSE, "output XON/XOFF"=FALSE, "output HW Handshake"=FALSE, "output alt HW HShk"=FALSE, "XOFF byte"=13, "XON byte"=11, "parity error byte"=0}, "parity"=w43, "buffer size"=w42, "stop bits"=w39, "data bits"=w40, "baud rate"=w41, "port number"=w38) -> ("error code"=w37:i32)
  n175 = call "CM Serial Port Setup.vi"("COM port"=w31, "time delay"=w32) -> ("time delay1"=w27:u32, "DK port Out"=w28:T1, "error code"=w30:i32)  [unwired: 7 in]
  n176 = Equal To 0?(x=w30) -> (x = 0?=w29:bool)
  n177 = Concatenate Strings("\r", "\n") -> (w33:string)
  n178 = while {
    tunnel: w38 -> [w479]
    tunnel: w33 -> [w480]
    tunnel: w37 -> [_]
    tunnel: "Axis" -> [w477]
    stop <- TRUE continue-if-true
    w478 = u32 200  # timeout
    n179 = Format Into String(w477) -> (resulting string=w481:string)  [unwired: 3 in, 1 out]
    n180 = stacked-sequence {
      seq-local: [w486 _ _ _] -> [_ w497 _ _]
      seq-local: [w485 _ _ _] -> [_ w496 _ _]
      seq-local: [w487 _ _ _] -> [_ w498 _ _]
      seq-local: [w484 _ _ _] -> [_ w494 _ _]
      seq-local: [_ w497 _ _] -> [_ _ w507 _]
      seq-local: [_ w496 _ _] -> [_ _ w506 _]
      seq-local: [_ w498 _ _] -> [_ _ w508 _]
      seq-local: [_ w494 _ _] -> [_ _ w504 _]
      seq-local: [_ _ w507 _] -> [_ _ _ w520]
      seq-local: [_ _ w506 _] -> [_ _ _ w517]
      seq-local: [_ _ w508 _] -> [_ _ _ w519]
      seq-local: [_ _ w504 _] -> [_ _ _ w518]
      tunnel: w481 -> [w486 _ _ _]
      tunnel: w480 -> [w485 _ _ _]
      tunnel: w479 -> [w487 _ _ _]
      tunnel: w478 -> [w484 _ _ _]
      frame #0 {
        n181 = case shown="False" "Motor ON" {
          tunnel: w487 -> [_ w493]
          tunnel: w486 -> [_ w490]
          tunnel: w485 -> [_ w489]
          frame False {
          }
          frame True {
            n182 = Concatenate Strings(w490, "MO" ("Substring"), w489) -> (w491:string)
            n183 = call <vilib>:"Serial Port Write.vi"("string to write"=w491, "port number"=w493) -> ()  [unwired: 1 out]
          }
        }
      }
      frame #1 {
        n184 = case shown="False" "Motor OFF" {
          tunnel: w498 -> [_ w503]
          tunnel: w497 -> [_ w500]
          tunnel: w496 -> [_ w499]
          frame False {
          }
          frame True {
            n185 = Concatenate Strings(w500, "MF" ("Substring"), w499) -> (w501:string)
            n186 = call <vilib>:"Serial Port Write.vi"("string to write"=w501, "port number"=w503) -> ()  [unwired: 1 out]
          }
        }
      }
      frame #2 {
        n187 = case shown="False" "Move" {
          tunnel: w508 -> [_ w515]
          tunnel: w507 -> [_ w512]
          tunnel: w506 -> [_ w511]
          frame False {
          }
          frame True {
            n188 = Format Into String("Target [mm]") -> (resulting string=w509:string)  [unwired: 3 in, 1 out]
            n189 = Concatenate Strings(w512, "PA" ("Substring"), w509, w511) -> (w513:string)
            n190 = call <vilib>:"Serial Port Write.vi"("string to write"=w513, "port number"=w515) -> ()  [unwired: 1 out]
          }
        }
      }
      frame #3 {
        n191 = case shown="False" "Set this as t0" {
          tunnel: w520 -> [_ w530]
          tunnel: w519 -> [_ w529]
          tunnel: w518 -> [_ w528]
          tunnel: w517 -> [_ w527]
          frame False {
          }
          frame True {
            n192 = flat-sequence {
              tunnel: w530 -> [w534]
              tunnel: w529 -> [w533]
              tunnel: [w533] -> w526
              tunnel: w528 -> [w531]
              tunnel: [w531] -> w525
              tunnel: w527 -> [w532]
              tunnel: w526 -> [w538]
              tunnel: [w538] -> w524
              tunnel: w525 -> [w537]
              tunnel: [w537] -> w523
              tunnel: [w539] -> w522
              tunnel: w524 -> [w544]
              tunnel: w523 -> [w542]
              tunnel: w522 -> [w541]
              tunnel: [w540] -> w521
              tunnel: w521 -> [w566]
              frame #0 {
                # "send position query"
                n193 = Concatenate Strings(w534, "TP" ("Substring"), w532) -> (w535:string)
                n194 = call <vilib>:"Serial Port Write.vi"("string to write"=w535, "port number"=w533) -> ()  [unwired: 1 out]
              }
              frame #1 {
                # "record current time"
                n195 = Tick Count (ms)() -> (millisecond timer value=w539:u32)
              }
              frame #2 {
                # "read characters in serial port"
                n196 = while {
                  shift-left: w541 -> [w545]
                  shift-right: [w546] -> _
                  tunnel: w542 -> [w549]
                  shift-left: "" -> [w552]
                  shift-right: [w551] -> w540
                  tunnel: w544 -> [w553]
                  stop <- w548 continue-if-true
                  n197 = Tick Count (ms)() -> (millisecond timer value=w547:u32)
                  n198 = call <vilib>:"Bytes At Serial Port.vi"("port number"=w553) -> ("byte count"=w554:u32)  [unwired: 1 out]
                  n199 = Subtract(x=w547, y=w545) -> (x-y=w550:u32)
                  n200 = Greater Than 0?(x=w554) -> (x > 0?=w555:bool)
                  n201 = case shown="True" w555 {
                    tunnel: w554 -> [_ w563]
                    tunnel: w553 -> [_ w562]
                    tunnel: w552 -> [w557 w560]
                    tunnel: [w557 w559] -> w551
                    tunnel: [w556 w558] -> w546
                    tunnel: w547 -> [_ w558]
                    tunnel: w545 -> [w556 _]
                    frame False {
                    }
                    frame True {
                      n202 = call <vilib>:"Serial Port Read.vi"("requested byte count"=w563, "port number"=w562) -> ("string read"=w561:string)  [unwired: 1 out]
                      n203 = Concatenate Strings(w560, w561) -> (w559:string)
                    }
                  }
                  n204 = Less?(x=w550, y=w549) -> (x < y?=w548:bool)
                }
              }
              frame #3 {
                n205 = Scan From String(input string=w566) -> (output 1=w564:dbl)  [unwired: 4 in, 3 out]
                n206 = Subtract(x=w564, y=w564) -> (x-y=→"Initial position [mm]":dbl)
              }
            }
          }
        }
      }
    }
    n207 = Wait Until Next ms Multiple(millisecond multiple=u32 50) -> ()  [unwired: 1 out]
  }
  n208 = case shown="True" w29 {
    tunnel: w28 -> [w569 w572]
    tunnel: w27 -> [w568 w571]
    tunnel: [w569 w572] -> w4
    tunnel: [w568 w571] -> w5
    tunnel: [TRUE FALSE] -> w3
    frame False {
    }
    frame True {
      n209 = call "CM Com Write ini.vi"("time delay1"=w572, "Mono port"=w571) -> ()  [unwired: 7 in]
      n210 = local write "Mono port"(w572) -> ()
      n211 = local write "Time delay"(w571) -> ()
    }
  }
  n212 = call "Configure.vi"("Dwell Time (s)"="Time between measurements\n at one point (s)/Dwell Time", "Channel T Input"="Trigger mode", "Channel B Input"="Channel B Input", "Channel A Input"="Channel A Input", "Integrating time, 10^-7 sec"="Integrating time \nin 10^-7 sec", "gate mode (CW:0)"="gate mode (CW:0)", "Scan End Mode"=FALSE, "Number of Periods"="Number of Measurements\n to take at one point/ Number of Periods", "Count Mode"="Count Mode", "GPIB Address"="GPIB address") -> ()
  n213 = case shown="False" "?" {
    tunnel: w5 -> [_ w574]
    tunnel: w4 -> [_ w573]
    frame False {
    }
    frame True {
      n214 = Two Button Dialog(message="Do you want to change grating?", 1:"No" ("F button name (\"Cancel\")"), 2:"Yes" ("T button name (\"OK\")")) -> (T button?=w575:bool)
      n215 = case shown="True" w575 {
        tunnel: w574 -> [_ w580]
        tunnel: w573 -> [_ w579]
        frame False {
        }
        frame True {
          n216 = Two Button Dialog(message="Disable voltage from PMT", 1:"Do not swich grating" ("F button name (\"Cancel\")"), 2:"Done" ("T button name (\"OK\")")) -> (T button?=w581:bool)
          n217 = case shown="True" w581 {
            tunnel: w580 -> [_ w599]
            tunnel: w579 -> [_ w598]
            frame False {
            }
            frame True {
              n218 = flat-sequence {
                tunnel: w599 -> [w603]
                tunnel: [w603] -> w596
                tunnel: w598 -> [w602]
                tunnel: [w602] -> w595
                tunnel: [w600] -> w594
                tunnel: w596 -> [w607]
                tunnel: [w607] -> w593
                tunnel: w595 -> [w608]
                tunnel: [w608] -> w592
                tunnel: w594 -> [w606]
                tunnel: [w606] -> w591
                tunnel: w593 -> [w614]
                tunnel: [w614] -> w590
                tunnel: w592 -> [w613]
                tunnel: [w613] -> w589
                tunnel: w591 -> [w611]
                tunnel: [w611] -> w588
                tunnel: w590 -> [w617]
                tunnel: [w617] -> w587
                tunnel: w589 -> [w618]
                tunnel: [w618] -> w586
                tunnel: w588 -> [w616]
                tunnel: [w616] -> w585
                tunnel: w587 -> [w622]
                tunnel: w586 -> [w623]
                tunnel: [w621] -> w597
                tunnel: w585 -> [w621]
                frame #0 {
                  n219 = local read "Grating #"() -> (w601:dbl)
                  n220 = case shown="2, Default" w601 {
                    tunnel: [1 2] -> w600
                    frame 2, Default {
                    }
                    frame 1 {
                    }
                  }
                  n221 = call "Select11x2.vi"("time delay"=w603, "NEW GRT?"=w600, "port number"=w602) -> ()  [unwired: 3 out]
                }
                frame #1 {
                  n222 = call "Goto11x.vi"("time delay"=w607, "WAVELENGTH"=u16 300, "port number"=w608) -> ()  [unwired: 3 out]
                }
                frame #2 {
                  n223 = call "Query11x.vi"("port number"=w613, "QUERY"=u16 0, "time delay"=w614) -> ("STATUS MESSAGE"=w610:u16)  [unwired: 3 out]
                  n224 = local write "Current wavelength"(w610) -> ()
                }
                frame #3 {
                  n225 = call "Query11x.vi"("port number"=w618, "QUERY"=u16 2, "time delay"=w617) -> ("STATUS MESSAGE"=w615:u16)  [unwired: 3 out]
                  n226 = local write "Grooves/mm"(w615) -> ()
                }
                frame #4 {
                  n227 = Divide(x=w622, y=i16 100 ("device (1)")) -> (x/y=w624:dbl)
                  n228 = call "Query11x.vi"("port number"=w623, "QUERY"=u16 3, "time delay"=w624) -> ("STATUS MESSAGE"=w620:u16)  [unwired: 3 out]
                  n229 = local write "Blaze angle"(w620) -> ()
                }
              }
              n230 = local write "Grating #"(w597) -> ()
            }
          }
        }
      }
    }
  }
  "Mono port" <- w31
  "Time delay" <- w32
